vi "USBTC08SetMainsFrequency.vi"(8 "error in (no error)":errorcluster, 9 "Mains Frequency":i16(ring) items=["50 Hz", "60 Hz"], 11 "Handle in":i16) -> (0 "error out":errorcluster, 3 "Handle out":i16)   [LabVIEW 2009]
uses:
  usbtc08.dll
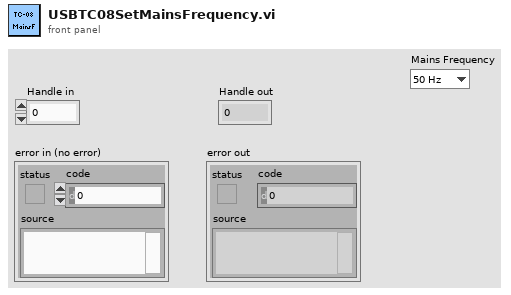
[diagram p1: front panel]
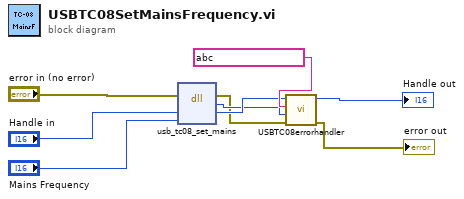
[diagram p0: block diagram]
diagram:
  n1 = dll-call lib="usbtc08.dll" fn="usb_tc08_set_mains" label="Set Mains"(error in="error in (no error)", "Handle"="Handle in", "sixtyHertz"="Mains Frequency") -> (error out=w2:errorcluster, "Return"=w4:i16, "Handle"=w5:i16)  [unwired: 3 in, 1 out]
  n2 = call "USBTC08errorhandler.vi"("error in (no error)"=w2, "Return"=w4, "API function"=string ?, "Handle in"=w5) -> ("error out"=→"error out":errorcluster, "Handle out"=→"Handle out":i16)  [unwired: 6 in]
